vi "getStructType.vi"(8 "error in (no error)":errorcluster, 11 "IStruct in":refnum<class "IStruct.lvclass">) -> (0 "error out":errorcluster, 2 "Struct Type out":refnum<class "IStructType.lvclass">, 3 "IStruct out":refnum<class "IStruct.lvclass">)   [LabVIEW 2022 SP3, in "openDAQ.lvlib" / "daqCoreTypes.lvlib" / "IStruct.lvclass"]
uses:
  <instrlib>/openDAQ/Public/Classes/daqCoreTypes/IStruct/IStruct.lvclass
  <instrlib>/openDAQ/Public/Classes/daqCoreTypes/IStruct/IStruct.lvclass/IStruct.ctl
  <instrlib>/openDAQ/Public/Classes/daqCoreTypes/IStructType/IStructType.lvclass
  <instrlib>/openDAQ/Binaries/Windows/x86/copendaq32.dll
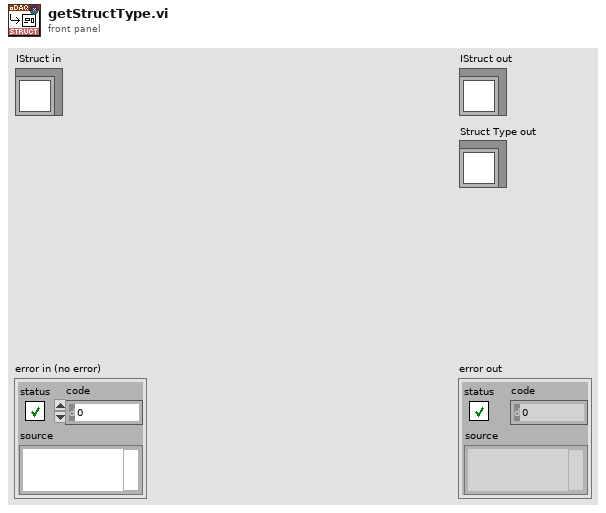
[diagram p1: front panel]
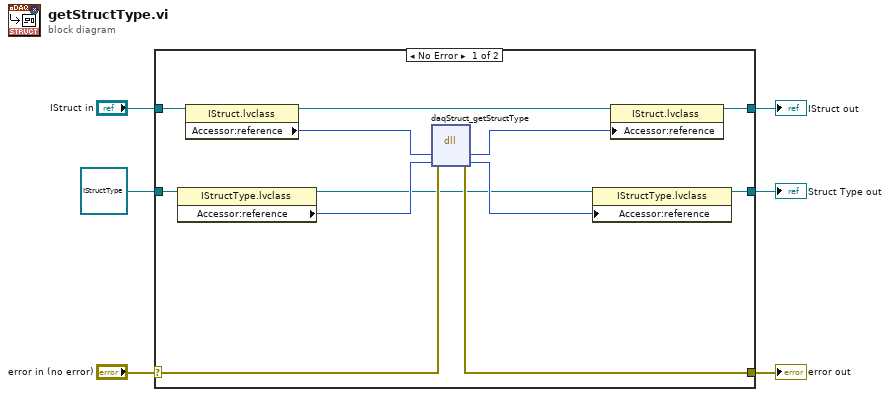
[diagram p0: block diagram]
diagram:
  n1 = case shown="No Error" "error in (no error)" {
    selector: "error in (no error)" -> [w16 w21]
    tunnel: [w15 w21] -> w5
    tunnel: [w10 w20] -> w3
    tunnel: "IStruct in" -> [w17 w20]
    tunnel: refnum<class "IStructType.lvclass"> refnum ("openDAQ.lvlib:IBaseObject.lvlib:IType.lvlib:IStructType.lvlib:IStructType.lvclass") -> [w14 w19]
    tunnel: [w8 w19] -> w1
    frame No Error {
      n2 = property class="IStructType.lvclass"(reference=w14) -> (reference out=w9:refnum<class "IStructType.lvclass">, "Accessor:reference"=w12:i64)  [unwired: 1 in, 1 out]
      n3 = property class="IStruct.lvclass"(reference=w17) -> (reference out=w11:refnum<class "IStruct.lvclass">, "Accessor:reference"=w13:i64)  [unwired: 1 in, 1 out]
      n4 = dll-call lib="C:/Program Files (x86)/National Instruments/LabVIEW 2022/instr.lib/openDAQ/Binaries/Windows/x86/copendaq*.*" fn="daqStruct_getStructType"(error in=w16, "struct"=w13, "structType"=w12) -> (error out=w15:errorcluster, "struct"=w7:i64, "structType"=w18:i64)  [unwired: 3 in, 1 out]
      n5 = property class="IStructType.lvclass"(reference=w9, "Accessor:reference"=w18) -> (reference out=w8:refnum<class "IStructType.lvclass">)  [unwired: 1 in, 1 out]
      n6 = property class="IStruct.lvclass"(reference=w11, "Accessor:reference"=w7) -> (reference out=w10:refnum<class "IStruct.lvclass">)  [unwired: 1 in, 1 out]
    }
    frame Error {
    }
  }
  "error out" <- w5
  "IStruct out" <- w3
  "Struct Type out" <- w1
